vi "BundleMessageCluster.vi"(8 "urgent? (F)":bool, 9 "atributes":variant, 10 "data":variant, 11 "name":string) -> (3 "message":T1)   [LabVIEW 2013, in "CLM_LocalMessage.lvclass"]
uses:
  CLM_LocalMessage.lvclass
  Message.ctl
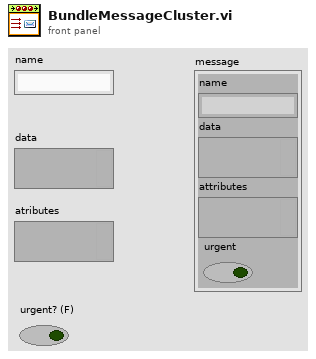
[diagram p1: front panel]
types:
  T1 = typedef "CLM_LocalMessage.lvclass/Message.ctl" = cluster{"name":string, "data":variant, "attributes":variant, "urgent":bool}
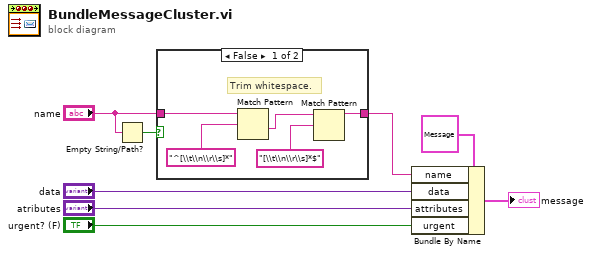
[diagram p0: block diagram]
diagram:
  n1 = Empty String/Path?(string/path="name") -> (empty?=w8:bool)
  n2 = case shown="False" w8 {
    tunnel: [w13 w14] -> w7
    tunnel: "name" -> [w9 w14]
    frame False {
      # "Trim whitespace."
      n3 = Match Pattern(string=w9, regular expression="^[\\t\\n\\r\\s]*") -> (after substring=w12:string)  [unwired: 1 in, 3 out]
      n4 = Match Pattern(string=w12, regular expression="[\\t\\n\\r\\s]*$") -> (before substring=w13:string)  [unwired: 1 in, 3 out]
    }
    frame True {
    }
  }
  n5 = Bundle By Name(cluster=T1 {"name"="", "data"=variant, "attributes"=variant, "urgent"=FALSE} ("message"), "name"=w7, "data"="data", "attributes"="atributes", "urgent"="urgent? (F)") -> (→"message":T1)
